vi "Add Server Library to Project.vi"(8 "error in (no error)":errorcluster, 10 "Project Settings":T1, 11 "Application in":refnum<vi>) -> (0 "error out":errorcluster)   [LabVIEW 2019, in "gRPC Scripting Tools.lvlib"]
uses:
  gRPC Scripting Tools.lvlib
  TypeDefs/Project Settings.ctl
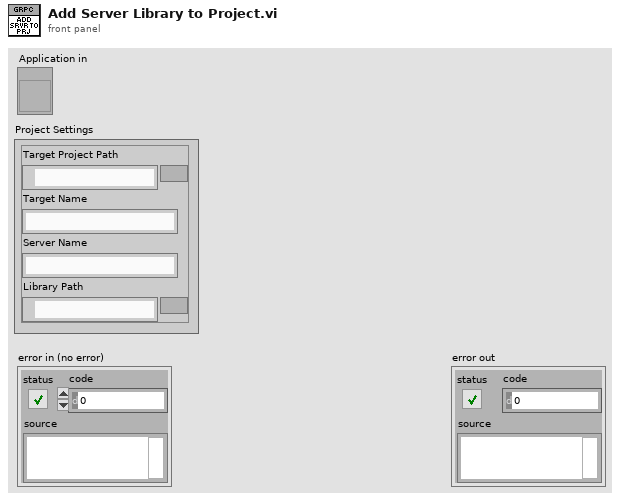
[diagram p1: front panel]
types:
  T1 = typedef "gRPC Scripting Tools.lvlib/Project Settings.ctl" = cluster{"Target Project Path":path, "Target Name":string, "Server Name":string, "Library Path":path}
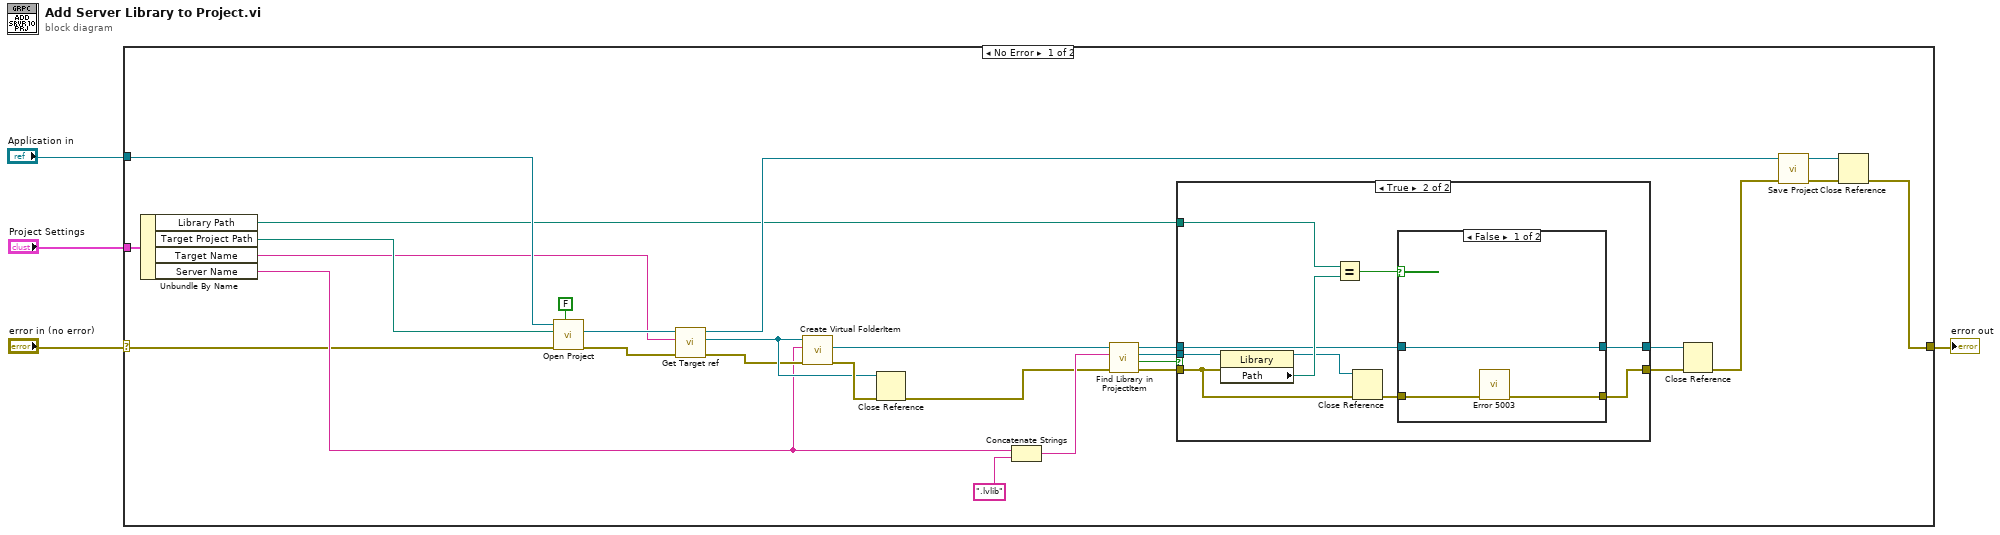
[diagram p0: block diagram]
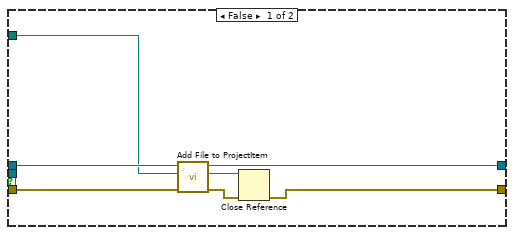
[diagram p2: hidden frame]
diagram:
  n1 = case shown="No Error" "error in (no error)" {
    selector: "error in (no error)" -> [w5 w55]
    tunnel: "Application in" -> [w23 _]
    tunnel: [w16 w55] -> w3
    tunnel: "Project Settings" -> [w10 _]
    frame No Error {
      n2 = Unbundle By Name(w10) -> ("Library Path"=w8:path, "Target Project Path"=w9:path, "Target Name"=w6:string, "Server Name"=w7:string)
      n3 = call "Open Project.vi"("Open Project Window ?"=FALSE, "error in (no error)"=w5, "Project Path in"=w9, "Application reference"=w23) -> ("error out"=w12:errorcluster, "Project out"=w15:refnum<vi>)  [unwired: 5 in, 1 out]
      n4 = call "Get Target ref.vi"("error in (no error)"=w12, "Target Name"=w6, "Project in"=w15) -> ("error out"=w11:errorcluster, "Target ref out"=w14:refnum<vi>, "Project out"=w13:refnum<vi>)  [unwired: 6 in]
      n5 = call "Create Virtual FolderItem.vi"("error in (no error)"=w11, "Folder Name"=w7, "ProjectItem in"=w14) -> ("error out"=w22:errorcluster, "FolderItem reference out"=w24:refnum<vi>)  [unwired: 5 in, 2 out]
      n6 = Close Reference(reference=w14, error in (no error)=w22) -> (error out=w19:errorcluster)
      n7 = Concatenate Strings(w7, ".lvlib" ("string")) -> (w26:string)
      n8 = call "Find Library in ProjectItem.vi"("error in (no error)"=w19, "Library Name"=w26, "ProjectItem in"=w24) -> ("error out"=w28:errorcluster, "Found?"=w27:bool, "Library out"=w30:refnum<vi>, "ProjectItem out"=w29:refnum<vi>)  [unwired: 5 in]
      n9 = case shown="True" w27 {
        tunnel: [w35 w45] -> w31
        tunnel: w28 -> [w36 w44]
        tunnel: w29 -> [w37 w47]
        tunnel: w30 -> [_ w43]
        tunnel: [w34 w46] -> w32
        tunnel: w8 -> [w33 w40]
        frame False {
          n10 = call "Add File to ProjectItem.vi"("error in (no error)"=w36, "File Path"=w33, "ProjectItem in"=w37) -> ("error out"=w38:errorcluster, "Added File ref"=w39:refnum<vi>, "ProjectItem out"=w34:refnum<vi>)  [unwired: 6 in]
          n11 = Close Reference(reference=w39, error in (no error)=w38) -> (error out=w35:errorcluster)
        }
        frame True {
          n12 = property class="Library"(reference=w43, error in=w44) -> (reference out=w41:refnum<vi>, "Path"=w49:path)  [unwired: 1 out]
          n13 = Equal?(x=w40, y=w49) -> (x = y?=w48:bool)
          n14 = Close Reference(reference=w41, error in (no error)=w44) -> (error out=w42:errorcluster)
          n15 = case shown="False" w48 {
            tunnel: w42 -> [w52 w53]
            tunnel: w47 -> [w51 w54]
            tunnel: [w51 w54] -> w46
            tunnel: [w50 w53] -> w45
            frame False {
              n16 = call "Error 5003.vi"("error in (no error)"=w52) -> ("error out"=w50:errorcluster)  [unwired: 10 in]
            }
            frame True {
            }
          }
        }
      }
      n17 = Close Reference(reference=w32, error in (no error)=w31) -> (error out=w20:errorcluster)
      n18 = call "Save Project.vi"("error in (no error)"=w20, "Project in"=w13) -> ("error out"=w18:errorcluster, "Project out"=w17:refnum<vi>)  [unwired: 8 in]
      n19 = Close Reference(reference=w17, error in (no error)=w18) -> (error out=w16:errorcluster)
    }
    frame Error {
    }
  }
  "error out" <- w3
